vi "LSP050Read.vi"(11 "voltage":dbl) -> (3 "level":dbl)   [LabVIEW 2020]
doc: "Converts voltage read at the output of the conditioning circuit of the LSP050 level transducer."
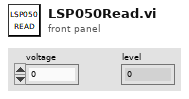
[diagram p1: front panel]
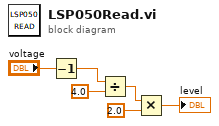
[diagram p0: block diagram]
diagram:
  n1 = Decrement(x="voltage") -> (x-1=w6:dbl)
  n2 = Divide(x=w6, y=4.0) -> (x/y=w2:dbl)
  n3 = Multiply(x=w2, y=2.0) -> (x*y=→"level":dbl)
